vi "Initialize Switch Action Processor.vi"(8 "error in (no error)":errorcluster, 9 "SLSC Device":refnum<k21>, 10 "SLSC Session In":refnum<class "SLSC Interface.lvclass">, 11 "Relays":refnum<class "Relay.lvclass">[](array[class])) -> (0 "error out":errorcluster, 3 "Switch Action Processor out":refnum<class "Switch Action Processor.lvclass">)   [LabVIEW 2016, in "SLSC Switch.lvlib" / "Switch Action Processor.lvclass"]
uses:
  Switch Action Processor.lvclass
  Relay/Relay.lvclass
  <vilib>/National Instruments/SLSC Local or Remote Interface/SLSC Interface Class/SLSC Interface.lvclass
  Switch Action Processor.lvclass/Switch Action Processor.ctl
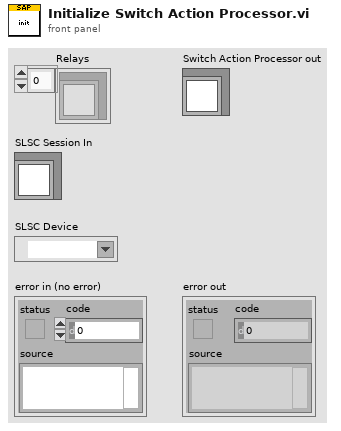
[diagram p1: front panel]
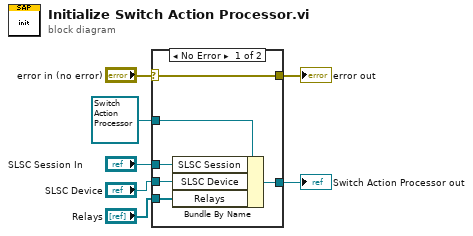
[diagram p0: block diagram]
diagram:
  n1 = case shown="No Error" "error in (no error)" {
    selector: "error in (no error)" -> [w13 w15]
    tunnel: [w13 w15] -> w6
    tunnel: [w11 w14] -> w4
    tunnel: refnum<class "Switch Action Processor.lvclass"> refnum ("Switch Action Processor in") -> [w12 w14]
    tunnel: "Relays" -> [w10 _]
    tunnel: "SLSC Session In" -> [w9 _]
    tunnel: "SLSC Device" -> [w8 _]
    frame No Error {
      n2 = Bundle By Name(cluster=w12, "SLSC Session"=w9, "SLSC Device"=w8, "Relays"=w10) -> (w11:refnum<class "Switch Action Processor.lvclass">)
    }
    frame Error {
    }
  }
  "error out" <- w6
  "Switch Action Processor out" <- w4
